vi "Begin.vi"() -> (0 "error out":errorcluster)   [LabVIEW 2015]
doc: "Called before other user functions, this VI is expected to open initial I/O refnums, load in file data, and do all program initialization. Notice that the <B>error out</B> terminal is simply used for data flow. Wiring it to other structures or subVIs ensures that this VI runs first."
uses:
  <vilib>/Rock Robotics/WPI/DriverStation/WPI_DriverStationRobotMode2.ctl
  DBNameEnum.ctl
  <vilib>/Rock Robotics/WPI/SafetyOutput/WPI_SafetyOutputConfigMenu.ctl
  <vilib>/Rock Robotics/WPI/Joystick/WPI_JoystickDeviceEnum.ctl
  RefnameEnum.ctl
  SingleSolenoidAction.ctl
  RollerAction.ctl
  TankDriveAction.ctl
  DoubleSolenoidAction.ctl
  CollectorAction.ctl
  <vilib>/Rock Robotics/WPI/Solenoid/WPI_SolenoidChannel.ctl
  <vilib>/Rock Robotics/SystemInterfaces/DIO/FPGA_DIOPWMChannel.ctl
  <vilib>/Rock Robotics/SystemInterfaces/Typedef/FPGA_TypedefDigitalModule.ctl
  <vilib>/Rock Robotics/SystemInterfaces/Typedef/FPGA_TypedefSolenoidModule.ctl
  <vilib>/Rock Robotics/SystemInterfaces/DIO/FPGA_DIOChannel.ctl
  <vilib>/Rock Robotics/SystemInterfaces/DIO/FPGA_DIORelayChannel.ctl
  <vilib>/Rock Robotics/WPI/Relay/WPI_RelayDirection.ctl
  <vilib>/Rock Robotics/SystemInterfaces/AI/FPGA_AIChannel.ctl
  SonarAction.ctl
  <vilib>/Rock Robotics/SystemInterfaces/Typedef/FPGA_TypedefAnalogModule.ctl
  Example_Code/PressureSensor/PressureSensorAction.ctl
  ServoAction.ctl
  LEDSaction.ctl
  Robot Global Data.vi
  <vilib>/Rock Robotics/WPI/Solenoid/WPI_SolenoidOpenSingle.vi
  <vilib>/Rock Robotics/WPI/MotorControl/WPI_MotorControlOpen Talon.vi
  <vilib>/Rock Robotics/WPI/Compressor/WPI_CompressorGetSetRefNum.vi
  <vilib>/Rock Robotics/WPI/RobotDrive/WPI_RobotDriveOpen4MotorWithTalon.vi
panel:
  in  "Version":string="TF 2.5.2"
  # "SET AS DEFAULT"
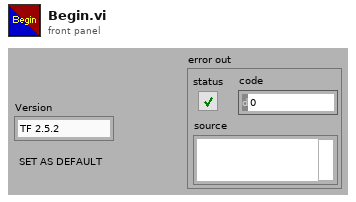
[diagram p1: front panel]
types:
  T1 = typedef "LEDSaction.ctl" = enum16{"Init", "10SecondsLeft", "LimitDown", "LimitUp", "CollectDown", "CollectUp", "NotHot", "Hot", "Shift", "RollBack", "RollFwd", "Shoot", "Distance Low", "DistanceHigh", "PressureLow", "PressureHigh"}
  T2 = typedef "FPGA_TypedefDigitalModule.ctl" = enum16{"Digital Module 1", "Digital Module 2"}
  T3 = typedef "ServoAction.ctl" = enum16{"Init", "SetAngle", "GetAngle", "Lower", "Raise", "Disable"}
  T4 = typedef "FPGA_DIOPWMChannel.ctl" = enum8{"PWM 1", "PWM 2", "PWM 3", "PWM 4", "PWM 5", "PWM 6", "PWM 7", "PWM 8", "PWM 9", "PWM 10", "Invalid"}
  T5 = typedef "PressureSensorAction.ctl" = enum16{"Init", "ReadValue", "Disable"}
  T6 = typedef "FPGA_AIChannel.ctl" = enum8{"AI 1", "AI 2", "AI 3", "AI 4", "AI 5", "AI 6", "AI 7", "AI 8", "Invalid"}
  T7 = typedef "FPGA_TypedefAnalogModule.ctl" = enum16{"Analog Module 1", "Analog Module 2"}
  T8 = typedef "FPGA_DIOChannel.ctl" = enum8{"DIO 1", "DIO 2", "DIO 3", "DIO 4", "DIO 5", "DIO 6", "DIO 7", "DIO 8", "DIO 9", "DIO 10", "DIO 11", "DIO 12", "DIO 13", "DIO 14", "Invalid"}
  T9 = typedef "SonarAction.ctl" = enum16{"Init", "ReadValue", "Disable"}
  T10 = typedef "WPI_RelayDirection.ctl" = enum16{"Both directions", "Forward only", "Reverse only"}
  T11 = typedef "FPGA_DIORelayChannel.ctl" = enum8{"Relay 1", "Relay 2", "Relay 3", "Relay 4", "Relay 5", "Relay 6", "Relay 7", "Relay 8", "Invalid"}
  T12 = typedef "WPI_SolenoidChannel.ctl" = enum8{"Solenoid 1", "Solenoid 2", "Solenoid 3", "Solenoid 4", "Solenoid 5", "Solenoid 6", "Solenoid 7", "Solenoid 8", "Invalid"}
  T13 = typedef "FPGA_TypedefSolenoidModule.ctl" = enum16{"Solenoid Module 1", "Solenoid Module 2"}
  T14 = typedef "SingleSolenoidAction.ctl" = enum16{"Init", "SetState", "Disable"}
  T15 = typedef "CollectorAction.ctl" = enum16{"Init", "Raise", "Lower", "Stop", "GetStatus"}
  T16 = typedef "DoubleSolenoidAction.ctl" = enum16{"Init", "Middle", "In", "Out"}
  T17 = typedef "TankDriveAction.ctl" = enum16{"Init", "LinearDrive", "SetValue", "Disable"}
  T18 = typedef "RefnameEnum.ctl" = enum16{"TankDrive", "Controller1", "Controller2", "SonicShifter", "Compressor"}
  T19 = typedef "RollerAction.ctl" = enum16{"Init", "Off", "Forward", "Reverse"}
  T20 = typedef "WPI_JoystickDeviceEnum.ctl" = enum16{"USB 0", "USB 1", "USB 2", "USB 3", "USB 4", "USB 5"}
  T21 = typedef "WPI_SafetyOutputConfigMenu.ctl" = enum16{"Enable", "Disable"}
  T22 = typedef "DBNameEnum.ctl" = enum16{"Version"}
  T23 = typedef "WPI_DriverStationRobotMode2.ctl" = enum16{"Autonomous Disabled", "Autonomous Enabled", "Teleop Disabled", "Teleop Enabled", "Disconnected", "Finish", "Test Disabled", "Test Enabled"}
  T24 = typedef "WPI_JoystickDevRef.ctl" = cluster{"Device":T20}
  T25 = typedef "WPI_RobotDriveDevRef.ctl" = cluster{"DevStatus":errorcluster, "Motors[]":T26[], "Square Inputs":bool, "Max Output":dbl}
  T26 = typedef "WPI_MotorControlDeviceRef.ctl" = cluster{"DeviceStatus":errorcluster, "Type":enum16{"PWM", "CAN"}, "PWM":cluster{"Digital Module":T2, "PWM Channel":T4, "DeadBand":T27}, "CAN":cluster{"Device Number":u8, "Control Mode":T28, "Semaphore":T29, "Max Vout":dbl}, "Invert":bool, "TransformRef":T30, "InvTransformRef":T30}
  T27 = typedef "WPI_PWMDeadband.ctl" = cluster{"Name":string, "maxPositivePwm":i32, "minPositivePwm":i32, "centerPwm":i32, "maxNegativePwm":i32, "minNegativePwm":i32, "angularRange":u16}
  T28 = typedef "WPI_CANJaguar_ControlMode.ctl" = enum8{"Percent VBus", "Current", "Speed", "Position", "Voltage"}
  T29 = typedef "Semaphore RefNum" = refnum<k1>
  T30 = typedef "WPI_PWMTransform_ConPane.ctl" = refnum<vi>
  T31 = typedef "WPI_SolenoidDevRef.ctl" = cluster{"DevStatus":errorcluster, "Solenoid Module":T13, "Forward Solenoid Channel":T12, "Reverse Solenoid Channel":T12}
  T32 = typedef "WPI_AnalogChannelDevRef.ctl" = cluster{"DevStatus":errorcluster, "Analog Module":T7, "Analog Channel":T6}
  T33 = typedef "WPI_DigitalInputDevRef.ctl" = cluster{"DevStatus":errorcluster, "DIO Channel":T8, "Digital Module":T2}
  T34 = typedef "WPI_CompressorDevRef.ctl" = cluster{"DevStatus":errorcluster, "DigitalInputDevRef":T33, "RelayDevRef":T35}
  T35 = typedef "WPI_RelayDevRef.ctl" = cluster{"DevStatus":errorcluster, "Relay Channel":T11, "Digital Module":T2, "Relay Direction":T10}
  T36 = typedef "WPI_ServoDeviceRef.ctl" = cluster{"DeviceStatus":errorcluster, "Digital Module":T2, "PWM Channel":T4, "DeadBand":T27}
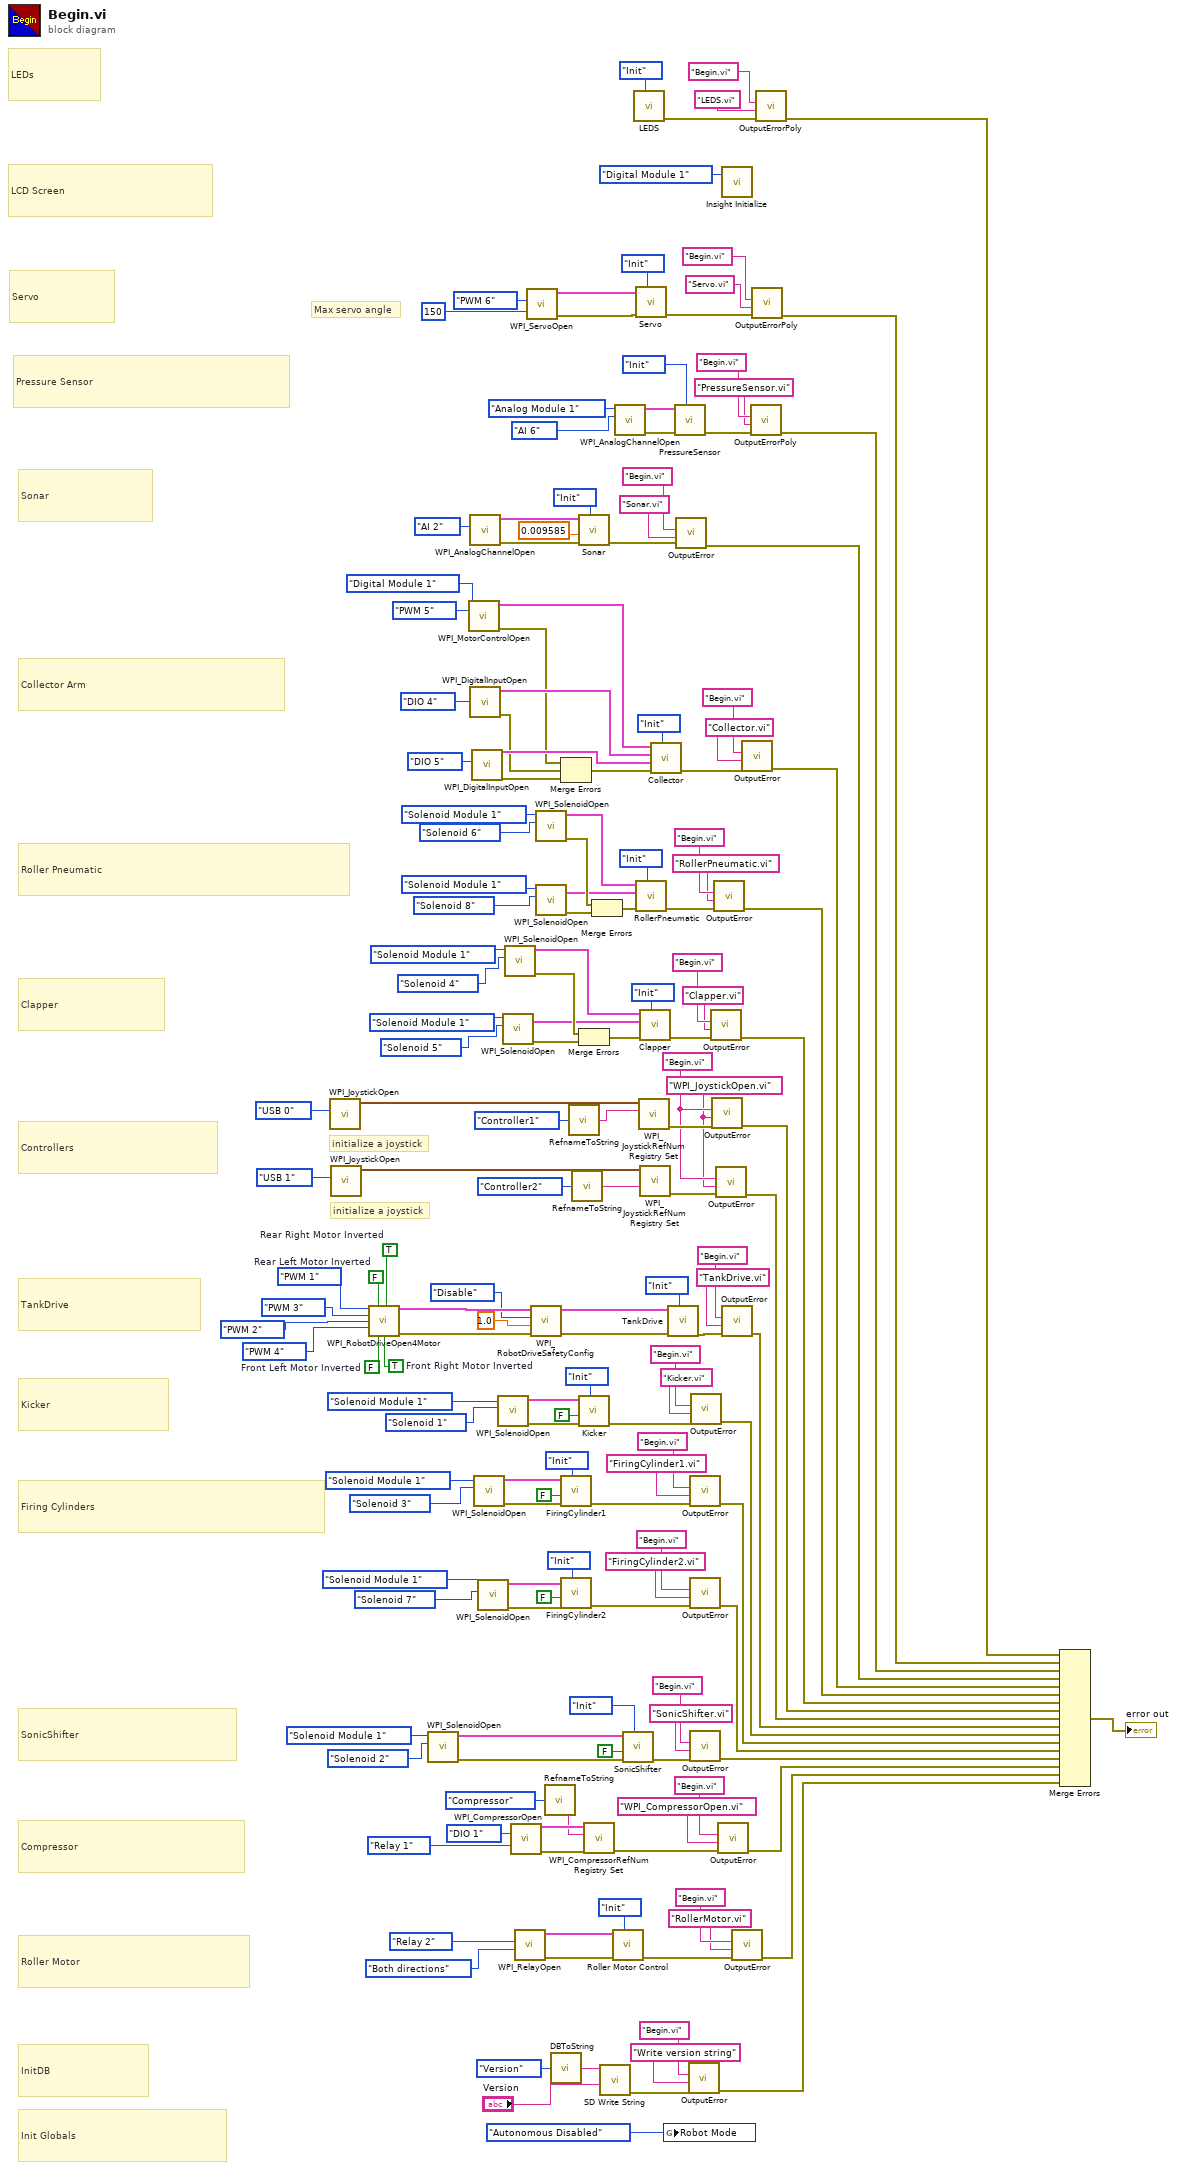
[diagram p0: block diagram]
diagram:
  w30 = TRUE  # Front Right Motor Inverted
  w31 = FALSE  # Front Left Motor Inverted
  w32 = TRUE  # Rear Right Motor Inverted
  w33 = FALSE  # Rear Left Motor Inverted
  w159 = "WPI_JoystickOpen.vi" ("Causing VI")
  w160 = "Begin.vi" ("Calling VI")
  # "LEDs"
  # "Max servo angle"
  # "LCD Screen"
  # "Servo"
  # "Pressure Sensor"
  # "Sonar"
  # "Collector Arm"
  # "Firing Cylinders"
  # "Roller Pneumatic"
  # "Clapper"
  # "Compressor"
  # "Roller Motor"
  # "SonicShifter"
  # "Controllers"
  # "initialize a joystick"
  # "initialize a joystick"
  # "TankDrive"
  # "Init Globals"
  # "InitDB"
  # "Kicker"
  n1 = call <vilib>:"WPI_JoystickOpen.vi"("JoystickDevice"=WPI_JoystickDeviceEnum."USB 0") -> ("JoystickDevRef"=w168:T24)  [unwired: 10 in]
  n2 = call <vilib>:"WPI_JoystickOpen.vi"("JoystickDevice"=WPI_JoystickDeviceEnum."USB 1") -> ("JoystickDevRef"=w165:T24)  [unwired: 10 in]
  n3 = call-poly <vilib>:"WPI_RobotDriveOpen4Motor.vi"("Rear Left Motor"=FPGA_DIOPWMChannel."PWM 1", "Rear Left Motor Inverted"=w33, "Rear Right Motor Inverted"=w32, "Rear Right Motor"=FPGA_DIOPWMChannel."PWM 3", "Front Left Motor"=FPGA_DIOPWMChannel."PWM 2", "Front Right Motor"=FPGA_DIOPWMChannel."PWM 4", "Front Left Motor Inverted"=w31, "Front Right Motor Inverted"=w30) -> ("RobotDriveDevRef"=w173:T25, "error out"=w172:errorcluster)  [unwired: 6 in]
  n4 = call-poly <vilib>:"WPI_SolenoidOpen.vi"("Solenoid Channel"=WPI_SolenoidChannel."Solenoid 2", "Solenoid Module (Module 1)"=FPGA_TypedefSolenoidModule."Solenoid Module 1") -> ("error out"=w116:errorcluster, "SolenoidDevRef"=w115:T31)  [unwired: 8 in]
  n5 = call-poly <vilib>:"WPI_MotorControlOpen.vi"("PWM Channel"=FPGA_DIOPWMChannel."PWM 5", "Digital Module (Module 1)"=FPGA_TypedefDigitalModule."Digital Module 1") -> ("error out"=w91:errorcluster, "MotorControlDeviceRef"=w97:T26)  [unwired: 8 in]
  n6 = call <vilib>:"WPI_AnalogChannelOpen.vi"("Analog Channel"=FPGA_AIChannel."AI 2") -> ("error out"=w45:errorcluster, "AIDeviceRef"=w46:T32)  [unwired: 9 in]
  n7 = call <vilib>:"WPI_DigitalInputOpen.vi"("DIO Channel"=FPGA_DIOChannel."DIO 4") -> ("error out"=w92:errorcluster, "DigitalInputDevRef"=w96:T33)  [unwired: 9 in]
  n8 = call <vilib>:"WPI_DigitalInputOpen.vi"("DIO Channel"=FPGA_DIOChannel."DIO 5") -> ("error out"=w93:errorcluster, "DigitalInputDevRef"=w95:T33)  [unwired: 9 in]
  n9 = call-poly <vilib>:"WPI_SolenoidOpen.vi"("Solenoid Channel"=WPI_SolenoidChannel."Solenoid 3", "Solenoid Module (Module 1)"=FPGA_TypedefSolenoidModule."Solenoid Module 1") -> ("error out"=w106:errorcluster, "SolenoidDevRef"=w105:T31)  [unwired: 8 in]
  n10 = call-poly <vilib>:"WPI_SolenoidOpen.vi"("Solenoid Channel"=WPI_SolenoidChannel."Solenoid 7", "Solenoid Module (Module 1)"=FPGA_TypedefSolenoidModule."Solenoid Module 1") -> ("error out"=w79:errorcluster, "SolenoidDevRef"=w78:T31)  [unwired: 8 in]
  n11 = call-poly <vilib>:"WPI_SolenoidOpen.vi"("Solenoid Channel"=WPI_SolenoidChannel."Solenoid 1", "Solenoid Module (Module 1)"=FPGA_TypedefSolenoidModule."Solenoid Module 1") -> ("error out"=w114:errorcluster, "SolenoidDevRef"=w111:T31)  [unwired: 8 in]
  n12 = call-poly <vilib>:"WPI_SolenoidOpen.vi"("Solenoid Channel"=WPI_SolenoidChannel."Solenoid 5", "Solenoid Module (Module 1)"=FPGA_TypedefSolenoidModule."Solenoid Module 1") -> ("error out"=w71:errorcluster, "SolenoidDevRef"=w70:T31)  [unwired: 8 in]
  n13 = call-poly <vilib>:"WPI_SolenoidOpen.vi"("Solenoid Channel"=WPI_SolenoidChannel."Solenoid 4", "Solenoid Module (Module 1)"=FPGA_TypedefSolenoidModule."Solenoid Module 1") -> ("error out"=w127:errorcluster, "SolenoidDevRef"=w126:T31)  [unwired: 8 in]
  n14 = call <vilib>:"WPI_CompressorOpen.vi"("Pressure Switch DIO Channel"=FPGA_DIOChannel."DIO 1", "Relay Channel"=FPGA_DIORelayChannel."Relay 1") -> ("CompressorDevRef"=w136:T34, "error out"=w135:errorcluster)  [unwired: 3 in, 9 out]
  n15 = call <vilib>:"WPI_RelayOpen.vi"("Relay Direction"=WPI_RelayDirection."Both directions", "Relay Channel"=FPGA_DIORelayChannel."Relay 2") -> ("error out"=w143:errorcluster, "RelayDevRef"=w141:T35)  [unwired: 8 in]
  n16 = call <vilib>:"WPI_ServoOpen.vi"("Angular Range"=u16 150, "PWM Channel"=FPGA_DIOPWMChannel."PWM 6") -> ("error out"=w16:errorcluster, "ServoDeviceRef"=w15:T36)  [unwired: 8 in]
  n17 = call <vilib>:"WPI_RobotDriveSafetyConfig.vi"("error in (no error)"=w172, "timeout (s)"=1.0, "mode"=WPI_SafetyOutputConfigMenu."Disable", "RobotDriveDevRef"=w173) -> ("error out"=w17:errorcluster, "RobotDriveDevRef"=w18:T25)  [unwired: 6 in]
  n18 = call-poly <vilib>:"WPI_SolenoidOpen.vi"("Solenoid Channel"=WPI_SolenoidChannel."Solenoid 6", "Solenoid Module (Module 1)"=FPGA_TypedefSolenoidModule."Solenoid Module 1") -> ("error out"=w117:errorcluster, "SolenoidDevRef"=w118:T31)  [unwired: 8 in]
  n19 = call-poly <vilib>:"WPI_SolenoidOpen.vi"("Solenoid Channel"=WPI_SolenoidChannel."Solenoid 8", "Solenoid Module (Module 1)"=FPGA_TypedefSolenoidModule."Solenoid Module 1") -> ("error out"=w66:errorcluster, "SolenoidDevRef"=w65:T31)  [unwired: 8 in]
  n20 = call "RefnameToString.vi"("Enum"=RefnameEnum."Compressor") -> ("Refname"=w133:string)
  n21 = call "DBToString.vi"("Enum"=DBNameEnum."Version") -> ("Refname"=w175:string)
  n22 = Merge Errors(w91, w92, w93) -> (w94:errorcluster)
  n23 = call "FiringCylinder1.vi"("Action"=SingleSolenoidAction."Init", "error in (no error)"=w106, "Default Position"=FALSE, "SolenoidDevRef"=w105) -> ("error out"=w107:errorcluster)  [unwired: 7 in]
  n24 = call "FiringCylinder2.vi"("Action"=SingleSolenoidAction."Init", "error in (no error)"=w79, "Default Position"=FALSE, "SolenoidDevRef"=w78) -> ("error out"=w74:errorcluster)  [unwired: 7 in]
  n25 = call "RefnameToString.vi"("Enum"=RefnameEnum."Controller1") -> ("Refname"=w157:string)
  n26 = call "RefnameToString.vi"("Enum"=RefnameEnum."Controller2") -> ("Refname"=w155:string)
  n27 = call "Sonar.vi"("Action"=SonarAction."Init", "error in (no error)"=w45, "Scaling factor (V/in)"=0.009585, "AIDeviceRef"=w46) -> ("error out"=w41:errorcluster)  [unwired: 6 in, 1 out]
  n28 = Merge Errors(w127, w71) -> (w72:errorcluster)
  n29 = call "Kicker.vi"("Action"=SingleSolenoidAction."Init", "error in (no error)"=w114, "Default Position"=FALSE, "SolenoidDevRef"=w111) -> ("error out"=w113:errorcluster)  [unwired: 7 in]
  n30 = call <vilib>:"WPI_CompressorRefNum Registry Set.vi"("error in (no error)"=w135, "refnum name"=w133, "CompressorDevRef"=w136) -> ("error out"=w6:errorcluster)  [unwired: 7 in, 1 out]
  n31 = Merge Errors(w117, w66) -> (w67:errorcluster)
  n32 = call <vilib>:"SD Write String.vi"("String"="Version", "Name"=w175) -> ("error out"=w152:errorcluster)  [unwired: 8 in, 1 out]
  n33 = call "Roller Motor Control.vi"("Action"=RollerAction."Init" ("RollerState"), "Error in"=w143, "RelayDevRef"=w141) -> ("Error out"=w142:errorcluster)  [unwired: 8 in]
  n34 = call <vilib>:"WPI_AnalogChannelOpen.vi"("Analog Channel"=FPGA_AIChannel."AI 6", "Analog Module (Module 1)"=FPGA_TypedefAnalogModule."Analog Module 1") -> ("error out"=w25:errorcluster, "AIDeviceRef"=w24:T32)  [unwired: 8 in]
  n35 = call "SonicShifter.vi"("Action"=SingleSolenoidAction."Init" ("Mode"), "error in (no error)"=w116, "Default Position"=FALSE, "SolenoidDevRef"=w115) -> ("error out"=w151:errorcluster)  [unwired: 7 in]
  n36 = call "LEDS.vi"("Action"=LEDSaction."Init") -> ("error out"=w4:errorcluster)  [unwired: 10 in]
  n37 = call "Servo.vi"("Action"=ServoAction."Init", "error in (no error)"=w16, "ServoDeviceRef"=w15) -> ("error out"=w12:errorcluster)  [unwired: 7 in, 1 out]
  n38 = call "RollerPneumatic.vi"("State"=DoubleSolenoidAction."Init", "Error in"=w67, "Plugged"=w65, "Open"=w118) -> ("Error out"=w121:errorcluster)  [unwired: 7 in]
  n39 = call <vilib>:"WPI_JoystickRefNum Registry Set.vi"("refnum name"=w157, "JoystickDevRef"=w168) -> ("error out"=w161:errorcluster)  [unwired: 8 in, 1 out]
  n40 = call "Clapper.vi"("State"=DoubleSolenoidAction."Init", "Error in"=w72, "Plugged"=w70, "Open"=w126) -> ("Error out"=w125:errorcluster)  [unwired: 7 in]
  n41 = call <vilib>:"WPI_JoystickRefNum Registry Set.vi"("refnum name"=w155, "JoystickDevRef"=w165) -> ("error out"=w162:errorcluster)  [unwired: 8 in, 1 out]
  n42 = call "Collector.vi"("Action"=CollectorAction."Init", "Error in"=w94, "BottomLS"=w95, "TopLS"=w96, "Motor"=w97) -> ("Error out"=w99:errorcluster)  [unwired: 4 in, 2 out]
  n43 = global write "Robot Global Data.vi" "Robot Mode"(WPI_DriverStationRobotMode2."Autonomous Disabled" ("Robot Mode")) -> ()
  n44 = call "TankDrive.vi"("DriveAction"=TankDriveAction."Init", "error in (no error)"=w17, "RobotDriveDevRef"=w18) -> ("error out"=w169:errorcluster)  [unwired: 7 in, 1 out]
  n45 = call "PressureSensor.vi"("Action"=PressureSensorAction."Init", "error in (no error)"=w25, "AIDeviceRef"=w24) -> ("error out"=w22:errorcluster)  [unwired: 7 in, 1 out]
  n46 = call "OutputError.vi"("error in (no error)"=w41, "Causing VI"="Sonar.vi", "Calling VI"="Begin.vi") -> ("error out"=w38:errorcluster)  [unwired: 8 in]
  n47 = call "OutputError.vi"("error in (no error)"=w152, "Causing VI"="Write version string", "Calling VI"="Begin.vi") -> ("error out"=w138:errorcluster)  [unwired: 8 in]
  n48 = call "OutputError.vi"("error in (no error)"=w107, "Causing VI"="FiringCylinder1.vi" ("Calling VI"), "Calling VI"="Begin.vi") -> ("error out"=w81:errorcluster)  [unwired: 8 in]
  n49 = call "OutputError.vi"("error in (no error)"=w74, "Causing VI"="FiringCylinder2.vi" ("Calling VI"), "Calling VI"="Begin.vi") -> ("error out"=w73:errorcluster)  [unwired: 8 in]
  n50 = call "OutputError.vi"("error in (no error)"=w151, "Causing VI"="SonicShifter.vi", "Calling VI"="Begin.vi") -> ("error out"=w150:errorcluster)  [unwired: 8 in]
  n51 = call "OutputError.vi"("error in (no error)"=w113, "Causing VI"="Kicker.vi" ("Calling VI"), "Calling VI"="Begin.vi") -> ("error out"=w82:errorcluster)  [unwired: 8 in]
  n52 = call "OutputError.vi"("error in (no error)"=w125, "Causing VI"="Clapper.vi", "Calling VI"="Begin.vi") -> ("error out"=w86:errorcluster)  [unwired: 8 in]
  n53 = call "OutputError.vi"("error in (no error)"=w161, "Causing VI"=w159, "Calling VI"=w160) -> ("error out"=w85:errorcluster)  [unwired: 8 in]
  n54 = call "OutputError.vi"("error in (no error)"=w121, "Causing VI"="RollerPneumatic.vi", "Calling VI"="Begin.vi") -> ("error out"=w87:errorcluster)  [unwired: 8 in]
  n55 = call "OutputError.vi"("error in (no error)"=w162, "Causing VI"=w159, "Calling VI"=w160) -> ("error out"=w84:errorcluster)  [unwired: 8 in]
  n56 = call "OutputError.vi"("error in (no error)"=w6, "Causing VI"="WPI_CompressorOpen.vi", "Calling VI"="Begin.vi") -> ("error out"=w132:errorcluster)  [unwired: 8 in]
  n57 = call "Insight Initialize.vi"("Digital Module"=FPGA_TypedefDigitalModule."Digital Module 1") -> ()  [unwired: 2 in]
  n58 = call "OutputError.vi"("error in (no error)"=w169, "Causing VI"="TankDrive.vi", "Calling VI"="Begin.vi") -> ("error out"=w83:errorcluster)  [unwired: 8 in]
  n59 = call "OutputError.vi"("error in (no error)"=w142, "Causing VI"="RollerMotor.vi", "Calling VI"="Begin.vi") -> ("error out"=w137:errorcluster)  [unwired: 8 in]
  n60 = call "OutputError.vi"("error in (no error)"=w99, "Causing VI"="Collector.vi", "Calling VI"="Begin.vi") -> ("error out"=w88:errorcluster)  [unwired: 8 in]
  n61 = call-poly "OutputErrorPoly.vi"("error in (no error)"=w22, "Causing VI"="PressureSensor.vi", "Calling VI"="Begin.vi") -> ("error out"=w21:errorcluster)  [unwired: 8 in]
  n62 = call-poly "OutputErrorPoly.vi"("error in (no error)"=w12, "Causing VI"="Servo.vi", "Calling VI"="Begin.vi") -> ("error out"=w9:errorcluster)  [unwired: 8 in]
  n63 = call-poly "OutputErrorPoly.vi"("error in (no error)"=w4, "Causing VI"="LEDS.vi", "Calling VI"="Begin.vi") -> ("error out"=w1:errorcluster)  [unwired: 8 in]
  n64 = Merge Errors(w1, w9, w21, w38, w88, w87, w86, w85, w84, w83, w82, w81, w73, w150, w132, w137, w138) -> (→"error out":errorcluster)
